vi "Publish Data.vi"(6 "Publish Time (Use Current Time)":timestamp, 8 "error in (no error)":errorcluster, 9 "Data to Publish":variant, 10 "Datum Name":string, 11 "IViewModel In":refnum<class "IViewModel.lvclass">) -> (0 "error out":errorcluster, 3 "IViewModel Out":refnum<class "IViewModel.lvclass">)   [LabVIEW 2017, in "IViewModel.lvlib" / "IViewModel.lvclass"]
doc: "<License>\nCopyright © 2017 Composed Systems, LLC | All rights reserved\nwww.composed.io\n\nAuthor: Ethan Stern <ethan.stern@composed.io>\n\nThis software is provided \"AS IS\" WITHOUT WARRANTIES, either express or implied, AND IS FOR EDUCATIONAL PURPOSES ONLY.\n</License>"
uses:
  IViewModel.lvclass
  C:/Git/mva-framework/Source/Framework/IObserver/IObserver/IObserver.lvclass
  <vilib>/ActorFramework/Actor/Actor.lvclass/Actor.ctl
  <vilib>/ActorFramework/Message Enqueuer/Message Enqueuer.lvclass/Message Enqueuer.ctl
  IMediator/PublishRequest/PublishRequest.lvclass/PublishRequest.ctl
  IViewModel.lvclass/IViewModel.ctl
  AbstractMessages/PreAddressedMsg/PreAddressedMsg.lvclass/PreAddressedMsg.ctl
  IMediator/IMediator Messages/Publish Msg/Publish Msg.lvclass/Publish Msg.ctl
  <vilib>/ActorFramework/Message Enqueuer/Enqueue.vi
  AbstractMessages/PreAddressedMsg/Read Return Address.vi
  <vilib>/ActorFramework/Actor/Read Self Enqueuer.vi
  <vilib>/ActorFramework/Message Enqueuer/Init from Existing Queue.vi
  IObserver/IObserver/IObserver.lvclass
  C:/Program Files (x86)/National Instruments/LabVIEW 2017/vi.lib/ActorFramework/Actor/Actor.lvclass
  IMediator/IMediator Messages/Publish Msg/Publish Msg.lvclass
  C:/Git/mva-framework/Source/Framework/AbstractMessages/PreAddressedMsg/PreAddressedMsg.lvclass
  C:/Program Files (x86)/National Instruments/LabVIEW 2017/vi.lib/ActorFramework/Message/Message.lvclass
  <vilib>/ActorFramework/Message Priority Queue/Priority Enqueue.vi
  IMediator/PublishRequest/PublishRequest.lvclass
  <vilib>/ActorFramework/Message Enqueuer/Message Enqueuer.lvclass
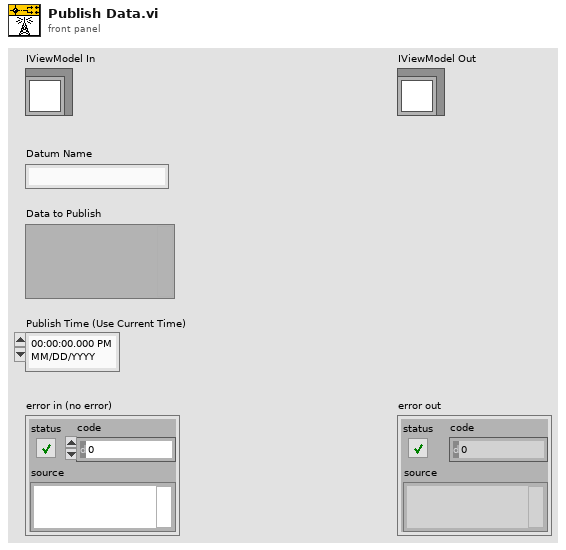
[diagram p1: front panel]
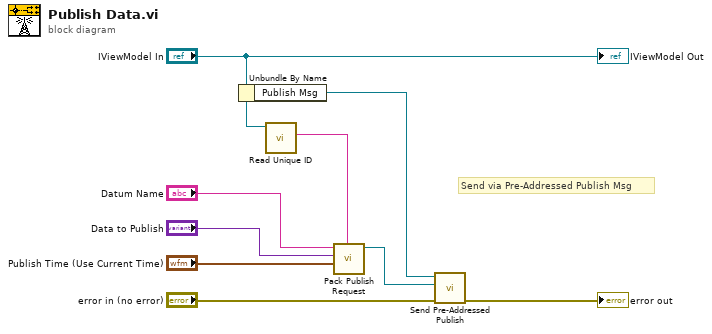
[diagram p0: block diagram]
diagram:
  # "Send via Pre-Addressed Publish Msg"
  n1 = Unbundle By Name("IViewModel In") -> ("Publish Msg"=w9:refnum<class "Publish Msg.lvclass">)
  n2 = call "Read Unique ID.vi"("IObserver In"="IViewModel In") -> ("Unique ID"=w1:string)  [unwired: 10 in]
  n3 = call "Pack Publish Request.vi"("Publisher ID"=w1, "Publish Time (Use Current Time)"="Publish Time (Use Current Time)", "Data to Publish"="Data to Publish", "Datum Name"="Datum Name") -> ("PublishRequest"=w4:refnum<class "PublishRequest.lvclass">)  [unwired: 7 in]
  n4 = call "Send Pre-Addressed Publish.vi"("error in (no error)"="error in (no error)", "PublishRequest"=w4, "Publish Message"=w9) -> ("error out"=→"error out":errorcluster)  [unwired: 8 in]
  "IViewModel Out" <- "IViewModel In"
